vi "Set Stream.vi"(8 "error in (no error)":errorcluster, 9 "Stream":refnum<class "Serial Stream.lvclass">, 10 "VISA resource name":refnum<visa-resource-name>, 11 "Serial Client in":refnum<class "Serial Client.lvclass">) -> (0 "error out":errorcluster, 3 "Serial Client out":refnum<class "Serial Client.lvclass">)   [LabVIEW 2020, in "Stream-Serial.lvlib" / "Serial Client.lvclass"]
uses:
  Serial Client.lvclass
  Serial Stream/Serial Stream.lvclass
  Serial Client.lvclass/Serial Client.ctl
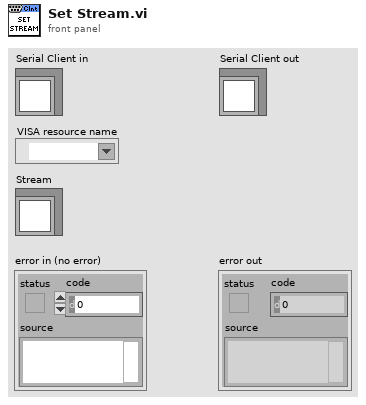
[diagram p1: front panel]
types:
  T1 = typedef "Stream-Serial.lvlib/Serial Client.lvclass/Ref Data.ctl" = cluster{"Stream":refnum<class "Serial Stream.lvclass">, "Client Loop":refnum<vi>, "Port Config":T2, "VISA Resource":refnum<visa-resource-name>}
  T2 = typedef "Stream-Serial.lvlib/Serial Client.lvclass/Port Config.ctl" = cluster{"Baud (115200)":u32, "Data Bits (8)":u8, "Stop Bits (1)":T3, "Flow Control":T4, "Use LineTerm?":bool, "LineTerm (\\n)":string, "Timeout ms (10000)":i32, "Parity (None)":T5}
  T3 = typedef "Stream-Serial.lvlib/Serial Client.lvclass/Stop Bits.ctl" = u16
  T4 = typedef "Stream-Serial.lvlib/Serial Client.lvclass/Flow Control.ctl" = u16
  T5 = typedef "Stream-Serial.lvlib/Serial Client.lvclass/Parity.ctl" = enum16{"None", "Odd", "Even", "Mark", "Space"}
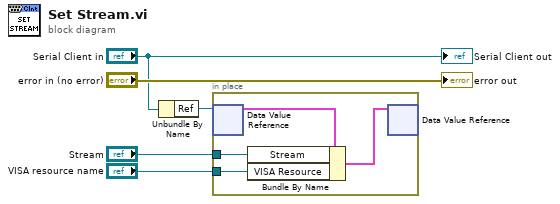
[diagram p0: block diagram]
diagram:
  n1 = Unbundle By Name("Serial Client in") -> ("Ref"=w4:refnum<data-value>)
  n2 = in-place {
    in-place-border: "Stream" -> [w7]
    in-place-border: "VISA resource name" -> [w6]
    n3 = in-place-dvr #1(w4) -> (w9:T1)  [unwired: 1 out]
    n4 = Bundle By Name(cluster=w9, "Stream"=w7, "VISA Resource"=w6) -> (w8:T1)
    n5 = in-place-dvr #1(w8) -> ()  [unwired: 2 out]
  }
  "error out" <- "error in (no error)"
  "Serial Client out" <- "Serial Client in"
